vi "odczyt pozycji TDMS.vi"() -> ()   [LabVIEW 2014]
uses:
  Kontrolki/FVGs/FVG akcje podstawowa.ctl
panel:
  in  "u¿yj x0 (T)":bool
  out "odczytane 2":dbl[][](graph)
  out "odczytane":dbl[][](graph)
  in  "file path":path
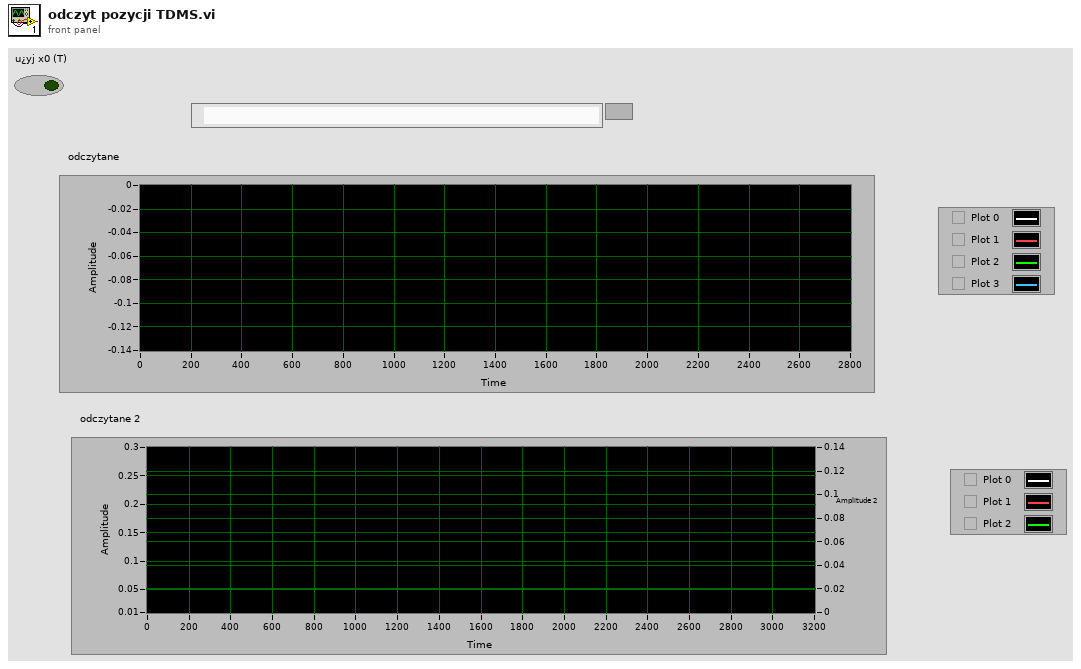
[diagram p1: front panel]
types:
  T1 = enum16{"open", "open or create", "create or replace", "create", "open (read-only)"}
  T2 = typedef "FVG akcje podstawowa.ctl" = enum16{"GET", "SET"}
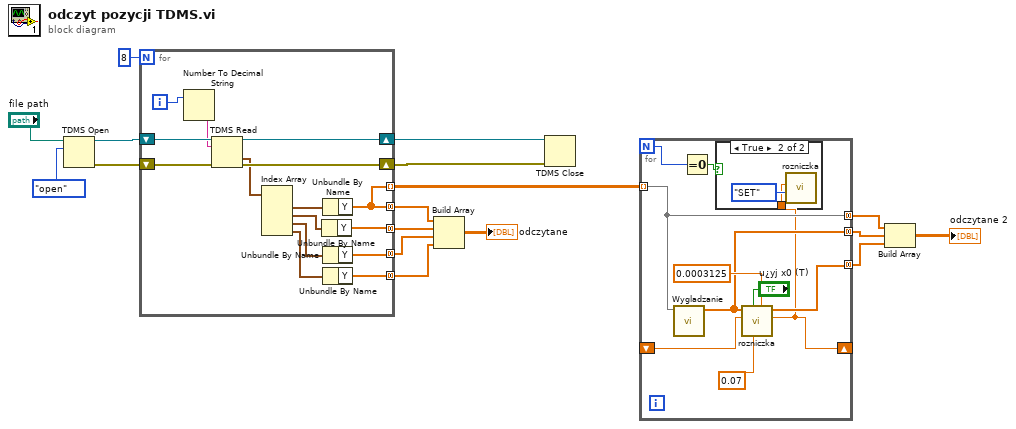
[diagram p0: block diagram]
diagram:
  n1 = TDMS Open(10:T1."open" ("operation (0:open)"), 11:"file path") -> (0:w14:errorcluster, 3:w15:refnum<k34>)  [unwired: 5 in]
  n2 = for {
    N: 8 -> [_]
    shift-right: [w29] -> w12
    shift-left: w15 -> [w32]
    shift-right: [w30] -> w13
    shift-left: w14 -> [w31]
    tunnel: [w18] -> w6 mode=concatenating
    tunnel: [w21] -> w10 mode=concatenating
    tunnel: [w20] -> w9 mode=concatenating
    tunnel: [w19] -> w8 mode=concatenating
    tunnel: [w18] -> w5 mode=indexing
    i -> [w28]
    n3 = Number To Decimal String(number=w28) -> (decimal integer string=w27:string)  [unwired: 1 in]
    n4 = TDMS Read(0:w32, 5:w27, 11:w31) -> (4:w29:refnum<k34>, 10:w26:waveform(dbl)[], 15:w30:errorcluster)  [unwired: 5 in, 3 out]
    n5 = Index Array(array=w26) -> (element #1=w25:waveform(dbl), element #2=w24:waveform(dbl), element #3=w23:waveform(dbl), element #4=w22:waveform(dbl))  [unwired: 4 in]
    n6 = Unbundle By Name(w24) -> ("Y"=w21:dbl[])
    n7 = Unbundle By Name(w25) -> ("Y"=w18:dbl[])
    n8 = Unbundle By Name(w23) -> ("Y"=w20:dbl[])
    n9 = Unbundle By Name(w22) -> ("Y"=w19:dbl[])
  }
  n10 = Build Array(w6, w10, w9, w8) -> (→"odczytane":dbl[][])
  n11 = TDMS Close(8:w13, 11:w12) -> ()  [unwired: 2 out]
  n12 = for {
    N -> [w33]
    tunnel: w5 -> [w40] mode=indexing
    tunnel: [w40] -> w4 mode=concatenating
    tunnel: [w39] -> w3 mode=concatenating
    tunnel: [w38] -> w2 mode=concatenating
    shift-right: [w35] -> _
    shift-left: _ -> [w36]
    n13 = call "Wygladzanie.vi"("Array in"=w40) -> ("Array out"=w39:dbl[])  [unwired: 10 in]
    n14 = Equal To 0?(x=w33) -> (x = 0?=w34:bool)
    n15 = call "rozniczka.vi"("dT"=0.0003125, 6:0.07 ("delta (0,7)"), "u¿yj x0 (T)"="u¿yj x0 (T)", "x0"=w36, "Array in"=w39) -> ("ostatni"=w35:dbl, "Array out"=w38:dbl[])  [unwired: 5 in]
    n16 = case shown="True" w34 {
      tunnel: w35 -> [_ w43]
      frame False {
      }
      frame True {
        n17 = call "rozniczka.vi"("Akcja (GET)"=FVG_akcje_podstawowa."SET", "x0"=w43) -> ()  [unwired: 8 in, 2 out]
      }
    }
  }
  n18 = Build Array(w4, w3, w2) -> (→"odczytane 2":dbl[][])
